vi "Write MsgString.vi"(8 "error in (no error)":errorcluster, 10 "MsgString":string, 11 "RealWorkActor in":refnum<class "RealWorkActor.lvclass">) -> (0 "error out":errorcluster, 3 "RealWorkActor out":refnum<class "RealWorkActor.lvclass">)   [LabVIEW 2021, in "RealWorkActor.lvlib" / "RealWorkActor.lvclass"]
uses:
  RealWorkActor.lvclass
  RealWorkActor.lvclass/RealWorkActor.ctl
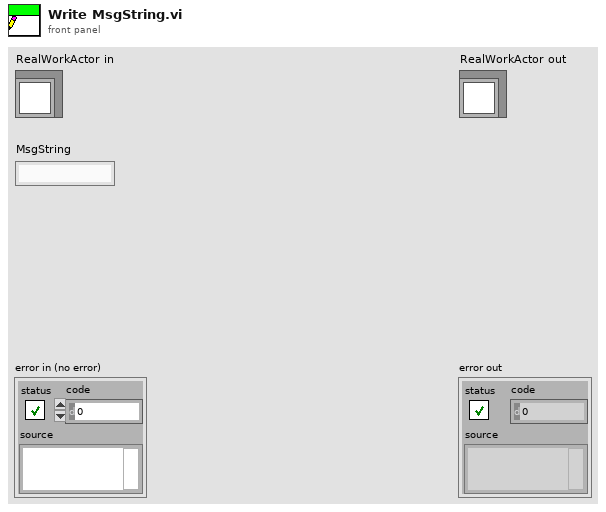
[diagram p1: front panel]
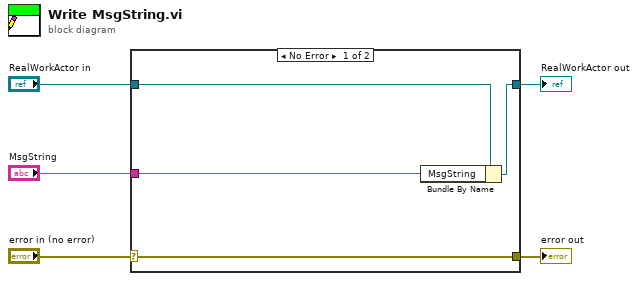
[diagram p0: block diagram]
diagram:
  n1 = case shown="No Error" "error in (no error)" {
    selector: "error in (no error)" -> [w9 w10]
    tunnel: [w9 w10] -> w4
    tunnel: [w7 w11] -> w2
    tunnel: "RealWorkActor in" -> [w8 w11]
    tunnel: "MsgString" -> [w6 _]
    frame No Error {
      n2 = Bundle By Name(cluster=w8, "MsgString"=w6) -> (w7:refnum<class "RealWorkActor.lvclass">)
    }
    frame Error {
    }
  }
  "error out" <- w4
  "RealWorkActor out" <- w2
